vi "3 and.vi"(1 "Boolean 3":bool, 2 "Boolean 2":bool, 3 "Boolean":bool) -> (0 "Boolean 4":bool)   [LabVIEW 2018]
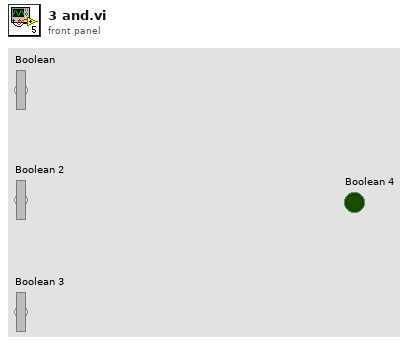
[diagram p1: front panel]
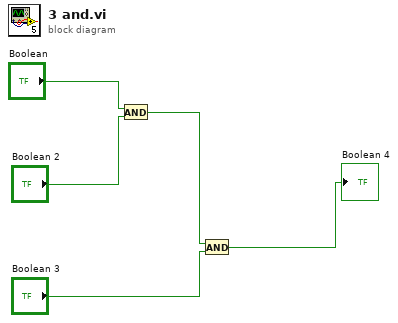
[diagram p0: block diagram]
diagram:
  n1 = And(x="Boolean", y="Boolean 2") -> (x .and. y?=w3:bool)
  n2 = And(x=w3, y="Boolean 3") -> (x .and. y?=→"Boolean 4":bool)
